vi "CheckStandAlrms.vi"(8 "error in (no error)":errorcluster, 11 "Stand in":refnum<class "Stand.lvclass">) -> (0 "error out":errorcluster, 3 "Stand out":refnum<class "Stand.lvclass">)   [LabVIEW 2019, in "Stand.lvclass"]
uses:
  Stand.lvclass
  D:/GIT H4000/H4000/src/Device_class/Device.lvclass
  Stand.lvclass/Stand.ctl
  DI_class/DI.lvclass/DI.ctl
  DA_class/DA.lvclass/DA.ctl
  Proccess_class/Proccess.lvclass/Proccess.ctl
  Device_class/Device.lvclass/Device.ctl
  subvis/bool_change.vi
  DA_class/private/write_to_db.vi
  Proccess_class/GetNames.vi
  Proccess_class/GetLogger.vi
  DA_class/DA.lvclass
  D:/GIT H4000/H4000/src/Proccess_class/Proccess.lvclass
  Logger_class/WriteEvent.vi
  FPGA_API_class/FPGA API.lvclass
  DI_class/DI.lvclass
  Device_class/Device.lvclass
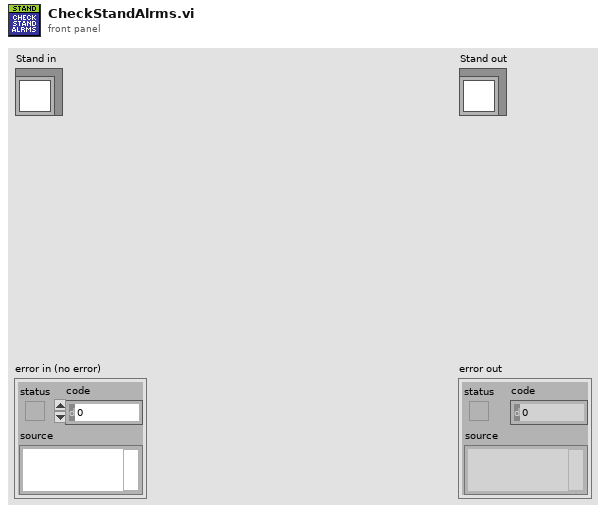
[diagram p1: front panel]
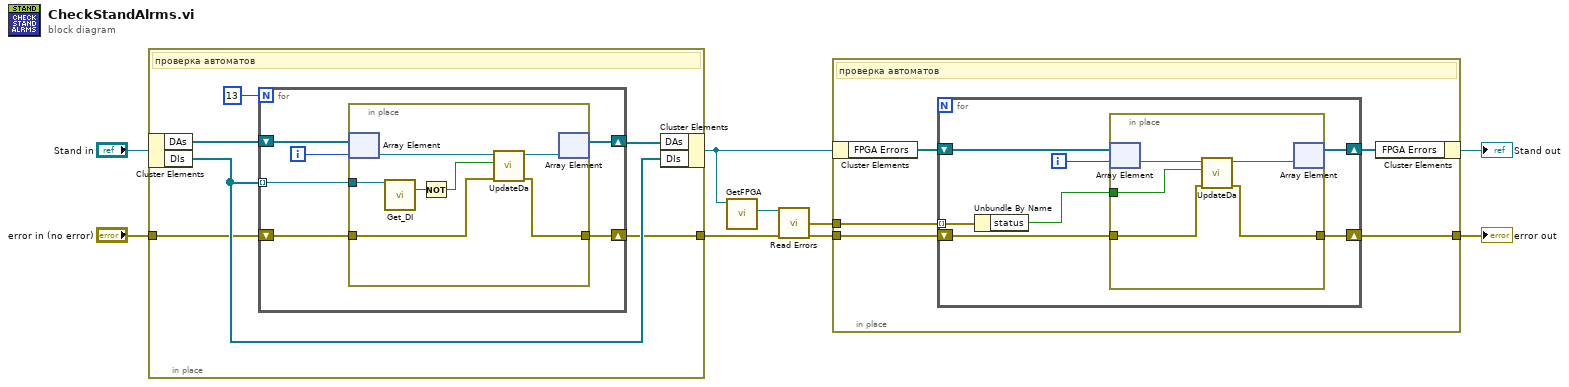
[diagram p0: block diagram]
diagram:
  n1 = in-place {
    in-place-border: "error in (no error)" -> [w11]
    in-place-border: [w10] -> w2
    # "проверка автоматов"
    n2 = in-place-cluster #1("Stand in") -> ("DAs"=w15:refnum<class "DA.lvclass">[], "DIs"=w12:refnum<class "DI.lvclass">[])
    n3 = for {
      N: 13 -> [_]
      tunnel: w12 -> [w21] mode=indexing
      shift-right: [w18] -> w14
      shift-left: w15 -> [w20]
      shift-right: [w16] -> w10
      shift-left: w11 -> [w17]
      i -> [w19]
      n4 = in-place {
        in-place-border: w21 -> [w28]
        in-place-border: w17 -> [w23]
        in-place-border: [w22] -> w16
        n5 = in-place-array #2(w20, w19) -> (w25:refnum<class "DA.lvclass">)
        n6 = call "Get_DI.vi"("reference in"=w28) -> ("DI"=w27:bool)  [unwired: 14 in]
        n7 = Not(x=w27) -> (.not. x?=w26:bool)
        n8 = call "UpdateDa.vi"("error in (no error)"=w23, "RAW"=w26, "Sig_DA in"=w25) -> ("error out"=w22:errorcluster, "Sig_DA out"=w24:refnum<class "DA.lvclass">)  [unwired: 6 in, 1 out]
        n9 = in-place-array #2(w24) -> (w18:refnum<class "DA.lvclass">[])  [unwired: 1 out]
      }
    }
    n10 = in-place-cluster #1("DAs"=w14, "DIs"=w12) -> (w8:refnum<class "Stand.lvclass">)
  }
  n11 = call "GetFPGA.vi"("Device in"=w8) -> ("FPGA API.lvclass"=w7:refnum<class "FPGA API.lvclass">)  [unwired: 10 in]
  n12 = call-dynamic "Read Errors.vi"("FPGA API in"=w7, "error in (no error)"=w2) -> ("Errors"=w6:errorcluster[], "error out"=w1:errorcluster)  [unwired: 11 in, 1 out]
  n13 = in-place {
    in-place-border: w6 -> [w31]
    in-place-border: w1 -> [w30]
    in-place-border: [w29] -> w3
    # "проверка автоматов"
    n14 = in-place-cluster #3(w8) -> ("FPGA Errors"=w33:refnum<class "DA.lvclass">[])
    n15 = for {
      shift-right: [w38] -> w32
      shift-left: w33 -> [w40]
      tunnel: w31 -> [w37] mode=indexing
      shift-right: [w34] -> w29
      shift-left: w30 -> [w35]
      i -> [w39]
      n16 = Unbundle By Name(w37) -> ("status"=w36:bool)
      n17 = in-place {
        in-place-border: w36 -> [w43]
        in-place-border: w35 -> [w42]
        in-place-border: [w41] -> w34
        n18 = in-place-array #4(w40, w39) -> (w45:refnum<class "DA.lvclass">)
        n19 = call "UpdateDa.vi"("error in (no error)"=w42, "RAW"=w43, "Sig_DA in"=w45) -> ("error out"=w41:errorcluster, "Sig_DA out"=w44:refnum<class "DA.lvclass">)  [unwired: 6 in, 1 out]
        n20 = in-place-array #4(w44) -> (w38:refnum<class "DA.lvclass">[])  [unwired: 1 out]
      }
    }
    n21 = in-place-cluster #3("FPGA Errors"=w32) -> (→"Stand out":refnum<class "Stand.lvclass">)
  }
  "error out" <- w3
